vi "BRig_Host__Loop_Producer__UploadClosedLoop__v4.vi"(1 "input_arrayBuffer_length":i32, 2 "input_arrayBuffer":u16[][](array[numeric]), 4 "input_cmdList":bool, 5 "input_cmdList":u16[][](array[numeric]), 6 "input_webdav_status":bool, 8 "session handle":T1, 9 "testNewLaserSettings":bool, 11 "input_array":u16[](array[numeric])) -> (12 "Sent":bool, 15 "output_arrayBuffer_length":i32, 16 "output_arrayBuffer":u16[][](array[numeric]))   [LabVIEW 2014]
uses:
  <vilib>/WebDAVClient/Advanced/SessionHandle.ctl
  <vilib>/Utility/file.llb/Write To Spreadsheet File (I64).vi
  <vilib>/WebDAVClient/Advanced/Put File.vi
  <vilib>/WebDAVClient/NI_WebDAV.lvlib
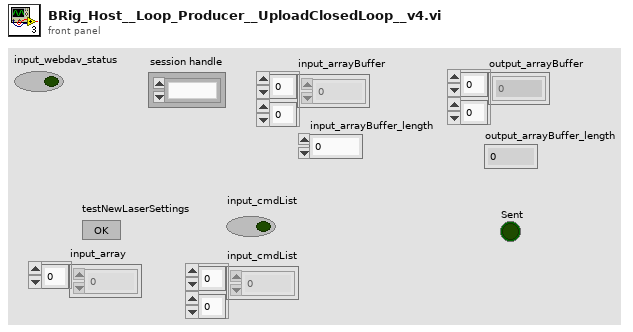
[diagram p1: front panel]
types:
  T1 = typedef "NI_WebDAV.lvlib/SessionHandle.ctl" = refnum<k1>
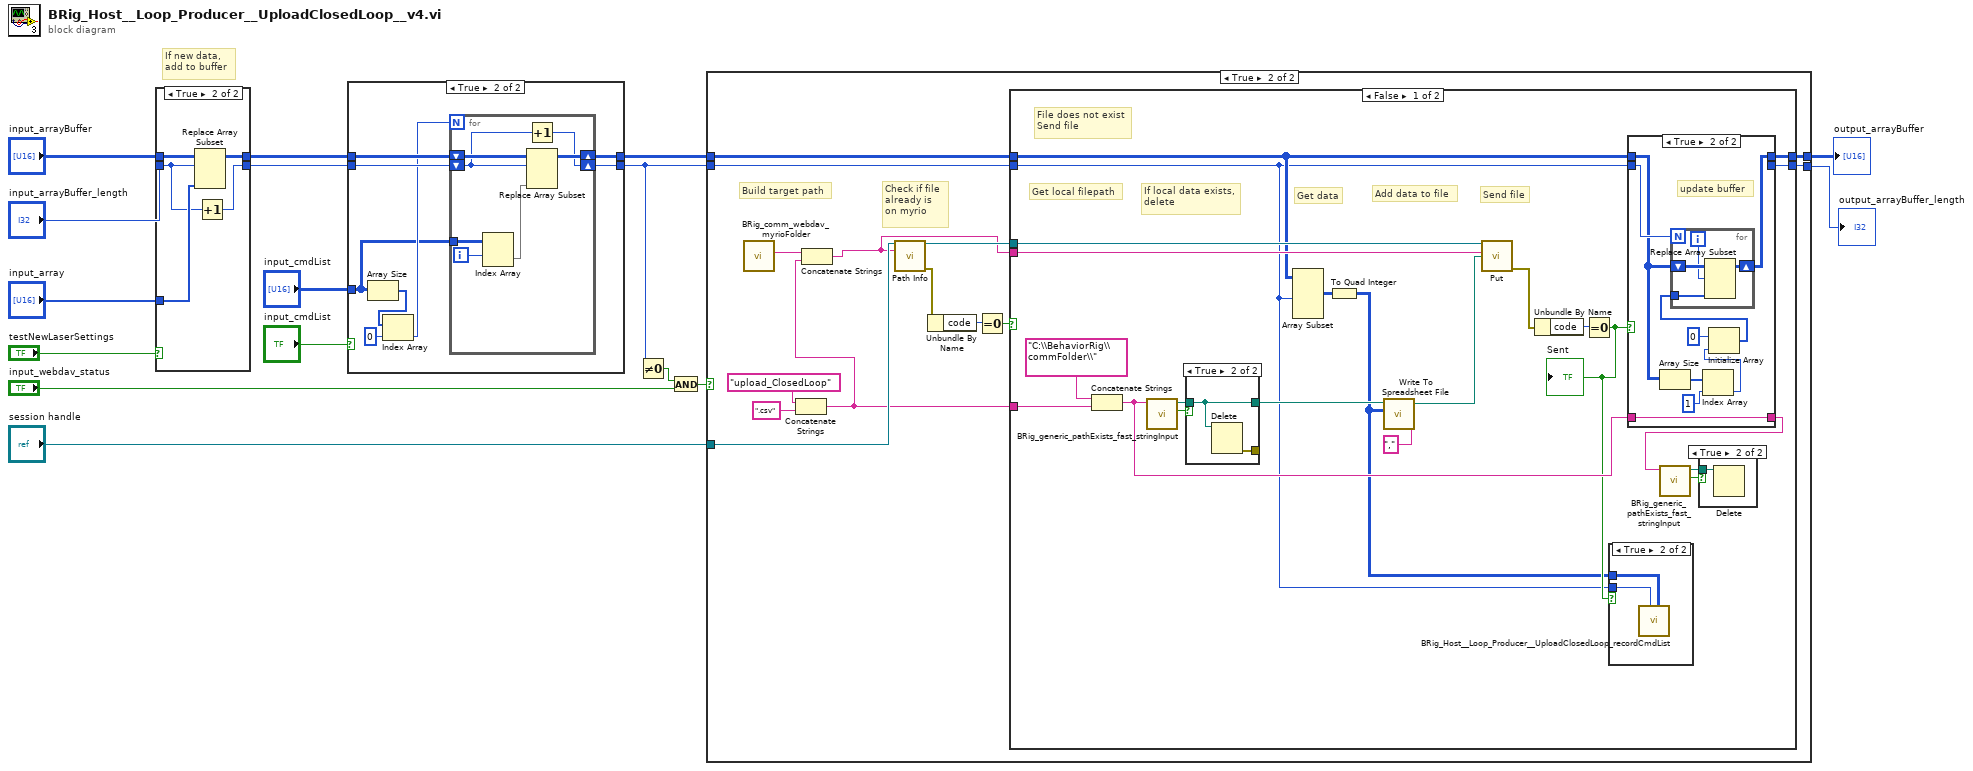
[diagram p0: block diagram]
diagram:
  # "If new data,\nadd to buffer"
  n1 = case shown="True" "testNewLaserSettings" {
    tunnel: "input_arrayBuffer" -> [w18 w23]
    tunnel: [w18 w21] -> w6
    tunnel: [w17 w19] -> w4
    tunnel: "input_arrayBuffer_length" -> [w17 w20]
    tunnel: "input_array" -> [_ w22]
    frame False {
    }
    frame True {
      n2 = Replace Array Subset(array=w23, new element=w22, index (row)=w20) -> (w21:u16[][])  [unwired: 1 in]
      n3 = Increment(x=w20) -> (x+1=w19:i32)
    }
  }
  n4 = case shown="True" "input_cmdList" {
    tunnel: w6 -> [w25 w31]
    tunnel: [w25 w30] -> w5
    tunnel: w4 -> [w24 w29]
    tunnel: [w24 w28] -> w3
    tunnel: "input_cmdList" -> [_ w26]
    frame False {
    }
    frame True {
      n5 = Array Size(array=w26) -> (size(s)=w33:i32[])
      n6 = Index Array(array=w33, index=0) -> (element=w27:i32)
      n7 = for {
        N: w27 -> [_]
        shift-right: [w37] -> w30
        shift-left: w31 -> [w38]
        shift-right: [w36] -> w28
        shift-left: w29 -> [w35]
        tunnel: w26 -> [w40]
        i -> [w39]
        n8 = Index Array(array=w40, index (row)=w39) -> (element=w34:u16[])  [unwired: 1 in]
        n9 = Increment(x=w35) -> (x+1=w36:i32)
        n10 = Replace Array Subset(array=w38, new element=w34, index (row)=w35) -> (w37:u16[][])  [unwired: 1 in]
      }
    }
  }
  n11 = Not Equal To 0?(x=w3) -> (x != 0?=w8:bool)
  n12 = And(x=w8, y="input_webdav_status") -> (x .and. y?=w7:bool)
  n13 = case shown="True" w7 {
    tunnel: "session handle" -> [_ w51]
    tunnel: w5 -> [w42 w49]
    tunnel: [w42 w48] -> w15
    tunnel: w3 -> [w41 w47]
    tunnel: [w41 w46] -> w14
    frame False {
    }
    frame True {
      # "Check if file\nalready is\non myrio"
      # "Build target path"
      n14 = call "BRig_comm_webdav_myrioFolder.vi"() -> ("output_myrioFolder"=w54:string)  [unwired: 11 in]
      n15 = Concatenate Strings("upload_ClosedLoop" ("string"), ".csv" ("string")) -> (w45:string)
      n16 = Concatenate Strings(w54, w45) -> (w43:string)
      n17 = call <vilib>:"Path Info.vi"("session handle"=w51, "relative uri"=w43) -> ("session handle out"=w44:T1, "error out"=w52:errorcluster)  [unwired: 10 in, 2 out]
      n18 = Unbundle By Name(w52) -> ("code"=w53:i32)
      n19 = Equal To 0?(x=w53) -> (x = 0?=w50:bool)
      n20 = case shown="False" w50 {
        tunnel: w49 -> [w70 w102]
        tunnel: [w69 w102] -> w48
        tunnel: w47 -> [w58 w101]
        tunnel: [w68 w101] -> w46
        tunnel: w45 -> [w78 _]
        tunnel: w44 -> [w72 _]
        tunnel: w43 -> [w71 _]
        frame False {
          # "Send file"
          # "Add data to file"
          # "Get data"
          # "If local data exists,\ndelete"
          # "Get local filepath"
          # "File does not exist\nSend file"
          n21 = Concatenate Strings("C:\\BehaviorRig\\commFolder\\", w78) -> (w64:string)
          n22 = call "BRig_generic_pathExists_fast_stringInput.vi"("input_filePath"=w64) -> ("output_Iexist"=w77:bool, "output_filePath"=w76:path)  [unwired: 8 in, 1 out]
          n23 = case shown="True" w77 {
            tunnel: w76 -> [w98 w99]
            tunnel: [_ w100] -> _
            tunnel: [w98 w99] -> w75
            frame False {
            }
            frame True {
              n24 = Delete(path (use dialog)=w99) -> (error out=w100:errorcluster)  [unwired: 4 in, 2 out]
            }
          }
          n25 = Array Subset(array=w70, length (row)=w58) -> (w61:u16[][])  [unwired: 3 in]
          n26 = To Quad Integer(1:w61) -> (0:w57:i64[][])
          n27 = call-poly <vilib>:"Write To Spreadsheet File.vi"("delimiter (\\t)"="," ("delimiter (\\t)"), "2D data"=w57, "file path (dialog if empty)"=w75) -> ("new file path (Not A Path if cancelled)"=w67:path)  [unwired: 5 in]
          n28 = call-poly <vilib>:"Put.vi"("session handle"=w72, "relative uri"=w71, "local file path"=w67) -> ("error out"=w74:errorcluster)  [unwired: 10 in, 2 out]
          n29 = Unbundle By Name(w74) -> ("code"=w73:i32)
          n30 = Equal To 0?(x=w73) -> (x = 0?=w59:bool)
          "Sent" <- w59
          n31 = case shown="True" w59 {
            tunnel: w58 -> [_ w80]
            tunnel: w57 -> [_ w79]
            frame False {
            }
            frame True {
              n32 = call "BRig_Host__Loop_Producer__UploadClosedLoop_recordCmdList.vi"("input_newData"=w79, "input_n"=w80) -> ()  [unwired: 10 in]
            }
          }
          n33 = case shown="True" w59 {
            tunnel: w70 -> [w84 w88]
            tunnel: [w84 w86] -> w69
            tunnel: w58 -> [w83 w93]
            tunnel: [w83 _] -> w68
            tunnel: w64 -> [w82 w85]
            tunnel: [w82 w85] -> w63
            frame False {
            }
            frame True {
              # "update buffer"
              n34 = Array Size(array=w88) -> (size(s)=w92:i32[])
              n35 = Index Array(array=w92, index=1) -> (element=w90:i32)
              n36 = Initialize Array(u16 0 ("element"), w90) -> (w87:u16[])
              n37 = for {
                N: w93 -> [_]
                shift-right: [w96] -> w86
                shift-left: w88 -> [w97]
                tunnel: w87 -> [w94]
                i -> [w95]
                n38 = Replace Array Subset(array=w97, new element=w94, index (row)=w95) -> (w96:u16[][])  [unwired: 1 in]
              }
            }
          }
          n39 = call "BRig_generic_pathExists_fast_stringInput.vi"("input_filePath"=w63) -> ("output_Iexist"=w65:bool, "output_filePath"=w66:path)  [unwired: 8 in, 1 out]
          n40 = case shown="True" w65 {
            tunnel: w66 -> [_ w81]
            frame False {
            }
            frame True {
              n41 = Delete(path (use dialog)=w81) -> ()  [unwired: 4 in, 3 out]
            }
          }
        }
        frame True {
          # "File does exist\nWait for myrio to process it"
        }
      }
    }
  }
  "output_arrayBuffer" <- w15
  "output_arrayBuffer_length" <- w14
